vi "set Defaults.vi"(0 "Session in":refnum<class "Test Number and Bin Generator.lvclass">=refnum, 11 "error in":errorcluster) -> (4 "Session out":refnum<class "Test Number and Bin Generator.lvclass">, 15 "error out":errorcluster)   [LabVIEW 2018, in "Test Number and Bin Generator.lvlib" / "Test Number and Bin Generator.lvclass"]
uses:
  Test Number and Bin Generator.lvclass
  Plugins/Sequence Automation Session.lvlibp/Sequence Automation Session.lvclass
  C:/Sequence Automation/Plugins/Sequence Automation Session.lvlibp/Sequence Automation Session.lvclass
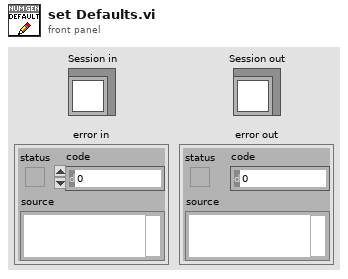
[diagram p1: front panel]
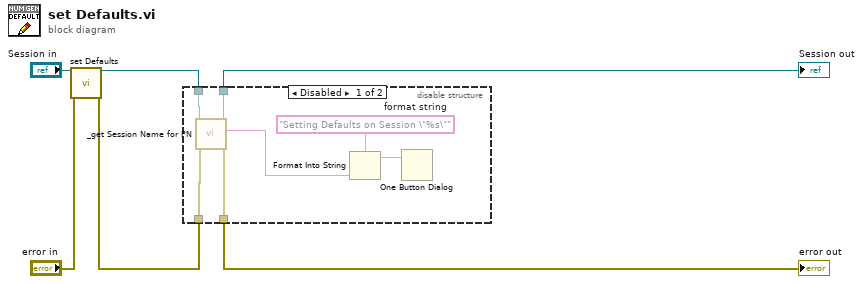
[diagram p0: block diagram]
diagram:
  n1 = call-parent "set Defaults.vi"("OBJ - Session in"="Session in", "error in"="error in") -> ("OBJ - Session out"=w3:refnum<class "Test Number and Bin Generator.lvclass">, "error out"=w1:errorcluster)  [unwired: 12 in]
  n2 = disable-structure shown="Disabled" {
    disable-tunnel: w3 -> [w13 w15]
    disable-tunnel: [w12 w15] -> w5
    disable-tunnel: w1 -> [w8 w14]
    disable-tunnel: [w7 w14] -> w6
    frame Disabled {
      w10 = "Setting Defaults on Session \"%s\""  # format string
      n3 = call "_get Session Name for PN.vi"("error in (no error)"=w8, "OBJ - Session in"=w13) -> ("error out"=w7:errorcluster, "Session Name"=w11:string, "OBJ - Session out"=w12:refnum<class "Test Number and Bin Generator.lvclass">)  [unwired: 7 in]
      n4 = Format Into String(format string=w10, w11) -> (resulting string=w9:string)  [unwired: 2 in, 1 out]
      n5 = One Button Dialog(message=w9) -> ()  [unwired: 1 in, 1 out]
    }
    frame Enabled {
    }
  }
  "error out" <- w6
  "Session out" <- w5
